vi "FestoCPX.Station.ProdSuctionGripper.Ready.vi"(7 "Log (T)":bool=TRUE, 8 "error in":errorcluster, 9 "Position":T1, 10 "Type":T2) -> (0 "error out":errorcluster, 2 "Ready state":T3)   [LabVIEW 2016]
uses:
  FestoCPX.Station.ProdSuctionGripper.ReadyState.ctl
  Station/Station.ProductSuctionGripper.Type.ctl
  Station/Station.ValvePosition.ctl
  tools/EventLog/EventLog.EventSource.ctl
  tools/Translator/Translator.Message.ctl
  tools/EventLog/EventLog.CreateError(array).vi
  tools/Translator/Translator.Translate.Status (NoError).vi
  tools/Translator/Translator.FormatMessage.vi
  tools/Translator/Translator.Global.vi
  tools/ErrorHandling/ErrorHandling.Create.vi
  Station/Station.Global.vi
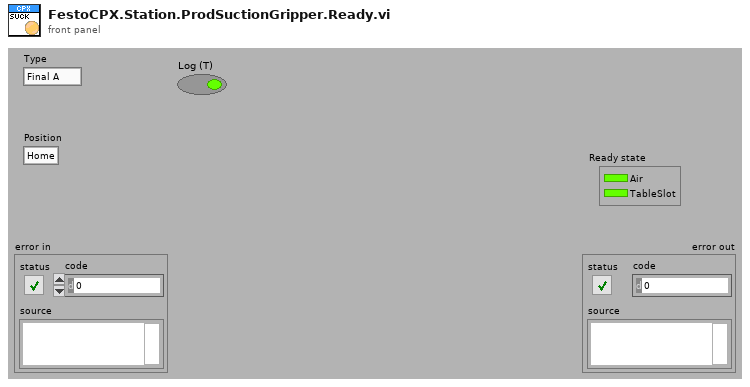
[diagram p1: front panel]
types:
  T1 = typedef "Station.ValvePosition.ctl" = enum16{"Home", "Work"}
  T2 = typedef "Station.ProductSuctionGripper.Type.ctl" = enum8{"Final A", "Final B", "Slot 1 A", "Slot 1 B", "Slot 2 A", "Slot 2 B", "Slot 3 A", "Slot 3 B", "Slot 4 A", "Slot 4 B"}
  T3 = typedef "FestoCPX.Station.ProdSuctionGripper.ReadyState.ctl" = cluster{"Air":bool, "TableSlot":bool}
  T4 = typedef "EventLog.EventSource.ctl" = enum16{"All", "Gui", "Ref", "File", "Arch", "Seq", "CPX", "DB", "Laser", "Scan.P", "Scan.O"}
  T5 = typedef "Translator.Message.ctl" = enum16{"-", "Event confirmed", "Log out", "Log in", "Shutdown", "Cancel", "Start", "Begin time", "End time", "Duration", "Service Mode", "Ignore Results", "Serial Format", "On", "Off", "OK", "NOK", "NOK %s", "Home", "Work", "Close", "Open", "In progress...", "Missing", "Empty", "Hardware failure", "Initial", "Default", "Total", "Out of range", "Free disk space is below 1GB - contact technician", "Error %d >> %s", "Error %d >> %s >> %s", "Msg %d >> %s", "Laser msg %d %s", "Laser cmd error %s %d", "Laser cmd failed %s", "Laser cmd warning %s", "Laser disconnected", "Laser status %s", "Laser already started", "Laser job unkonwn %s", "Laser job missing %s", "Laser job select failure %s", "Unable to start laser printing (%s)", "Unable to stop laser printing (%s)", "Laser marking aborted", "Laser marking timeout", "Unable to reset Laser Interlock (%s)", "Unable to trigger Laser. Laser not ready (%s)", "Laser job '%s' coordinates not configured", "Starting %s", "Quitting %s", "Configured", "Initializing", "Quitting", "Loading", "Loaded %d results", "Loaded %d events", "Running", "Stopped", "Summary", "Laser", "Do you want to continue?", "Do you want to delete the configuration?", "The configuration is being used by an order. Unable to delete!", "Press confirm button", "Station is not based. Do you want to exit?", "Station requires changeover. Do you want to run the test?", "Test options are not set as default. Do you want to continue?", "Formatting of WabcoNo is disabled. Do you want to continue?", "Product not detected. Do you want to continue?", "Product scan failed. Do you want to continue?", "Calibration", "Log out?", "System", "All", "IDLE", "Translating...%s", "Not found", "Alarm %s", "Run", "Skip", "Abort", "Repeat", "Please wait...", "Database disconnected", "Database disconnected - changeover disabled!", "Login to database successful", "Login to database failed: %d; %s", "Unable to check the product status of reference %d - database disconnected", "Unable to set the product status of reference %d - database disconnected", "Variant file backup %s", "Read variant (%s)", "Result", "Station armed!", "Station requires changeover!", "Select reference number...", "EMERGENCY BUTTON - press Control button", "EMERGENCY DOOR - press Control button", "Resetting Emergency...", "Unable to reset safety circuit - Emergency Button pressed", "Unable to reset safety circuit - Emergency Side Door open", "Station not based", "Station based", "Station not empty", "Station basing...", "No order", "Press Start to begin new order", "Scanning new order", "Order NOK. Correct or scan again", "Order OK. Press Accept", "Order ready", "Revolver incorrect", "Fork incorrect", "Revolver missing", "Revolver empty", "Container missing", "Offline results", "Offline statistics", "Updating statistics %.1f %%", "DMC Configurator", "Door open", "Close the front door", "Press start button", "Done. Open the front door", "Running...", "Running...%.1f %%", "Pause %s", "Pause %s. NOK container missing", "Pause %s. OK container missing", "Pause %s. Revolver empty", "Pause %s. Revolver missing", "Pause %s. Revolver incorrect", "Pause %s. Fork missing", "Pause %s. Fork incorrect", "Pause %s. Too many failures", "Pause %s. Unloading failure", "Pause %s. One slot is not working", "Pause %s. Part order is done. Empty OK container", "Pause %s. Unable to move product to slot", "Pause %s. Unable to move back product pusher", "Pause %s. Unable to lift product", "Pause %s. Unable to move back product lifter", "Pause %s. Unable to move product arm to Work", "Pause %s. Unable to move product arm to NOK", "Pause %s. Unable to move product arm to OK", "Pause %s. Unable to unsuck the NOK product", "Pause %s. Unable to drop the NOK product", "Pause %s. Product OK missing", "Pause %s. Unable to unsuck the OK product", "Pause %s. Unable to drop the OK product", "Stopping...", "File '%s' is missing", "File '%s' is broken", "File '%s' is running", "Log file started (%s)", "Log file ended (%s)", "Log file stopped (%s)", "Log file ignored (%s)", "Log file exported (%s)", "Log file export failed (%s)", "Wrong serial number in log file", "Wrong reference number in log file", "Test steps are missing", "%s = %.3f", "Process param '%s' not found in DB", "Process param '%s' wrong order", "Process param '%s' value %.3f out of limits (%.3f; %.3f)", "Step%d param '%s' not found in DB", "Step%d param '%s' wrong order", "Step%d param '%s' value %.3f out of limits (%.3f; %.3f)", "Step%d EV '%s' not found in DB", "Step%d EV '%s' wrong order", "\"%s\" not found in DB", "\"%s\" wrong order", "\"%s\" value %.3f out of limits (%.3f; %.3f)", "\"%s\" not found in software", "Process init (%s)", "Process started", "Process restarted", "Process run", "Process done", "Process done - remove OK container", "Process aborted", "Process aborted at work", "Process aborted at home", "Process error", "Process error at home", "Process error at work", "Process close", "Process pause", "Process continue", "Process door open", "Process door close", "Process pause at slot %s due to %s", "Select plate from the order to process", "Do you want to start the process?", "Do you want to continue the process?", "There is unfinished order. Do you want to put the new order?", "Product %s %d OK", "Product %s %d NOK", "Unable to unload the slot %s. Product missing in the slot", "Unable to unload the slot %s. Product already in the arm", "Unable to accept the product as OK. Product missing in slot %s", "Unable to accept the product as OK. Product could not drop into the container at slot %s", "Unable to accept the product as NOK. Product could not drop into the container at slot %s", "Scan failed. Error %s", "Scan failed. Scanner disconnected", "Scan failed. Wrong Wabco number %d, limit (%d,%d)", "Scan failed. Wrong serial number %d, limit (%d,%d)", "Scan failed. Wrong date %d, limit (%d,%d)", "Scan failed. Wrong product wabco number %d (expected %d)", "Scan failed. Wrong product serial number %d (expected > 0)", "Scan OK %s", "Scan failed. Unable to determine table position (%s)", "Scan failed. Timeout", "Tune failed. Scanner disconnected", "Tune failed. Timeout", "%s = %d", "%s = %d->%d", "Unable to set %s = %.2f - Air Pressure Inside off", "Unable to set digital output '%s' = %d", "Unable to activate air pressure inside - timeout", "Unable to activate air pressure inside - aborted", "Unable to switch on Air Main Valve - Air Pressure Inlet off", "Unable to switch on Air Main Valve - Door open", "Unable to switch off Air Main Valve - timeout", "Unable to switch off Air Main Valve - aborted", "Unable to rotate Table - timeout", "Unable to rotate Table - aborted", "Unable to rotate Table - Product Move not in Home position", "Unable to rotate Table - Air Pressure Inside off", "Unable to rotate Table - Product Lift A not in Home position", "Unable to rotate Table - Product Lift B not in Home position", "Unable to rotate Table - unlock before movement timeout", "Unable to rotate Table - lock after movement timeout", "Unable to move Table Lock to %s position - timeout", "Unable to move Table Lock to %s position - aborted", "Unable to move Table Lock to %s position - Air Pressure Inside off", "Unable to move Table Lock to %s position - Table not in position", "Unable to move Product Lift A to %s position - timeout", "Unable to move Product Lift B to %s position - timeout", "Unable to move Product Lift A to %s position - aborted", "Unable to move Product Lift B to %s position - aborted", "Unable to move Product Lift A to %s position - Air Pressure Inside off", "Unable to move Product Lift B to %s position - Air Pressure Inside off", "Unable to move Product Lift A to %s position - Table not locked", "Unable to move Product Lift B to %s position - Table not locked", "Unable to move Product Lift A to %s position - Product Arm not in Work position", "Unable to move Product Lift B to %s position - Product Arm not in Work position", "Unable to set Product Suction Gripper %s to %s - timeout", "Unable to set Product Suction Gripper %s to %s - aborted", "Unable to set Product Suction Gripper %s to %s - Air Pressure Inside off", "Unable to set Product Suction Gripper %s to %s - Table slot unkown", "Unable to move Product Arm to %s position - timeout", "Unable to move Product Arm to %s position - aborted", "Unable to move Product Arm to %s position - Air Pressure Inside off", "Unable to move Product Arm to %s position - Product Lift A not in Home position", "Unable to move Product Arm to %s position - Product Lift B not in Home position", "Unable to move Product to %s position - timeout", "Unable to move Product to %s position - aborted", "Unable to move Product to %s position - Air Pressure Inside off", "Unable to move Product to %s position - Table not in position"}
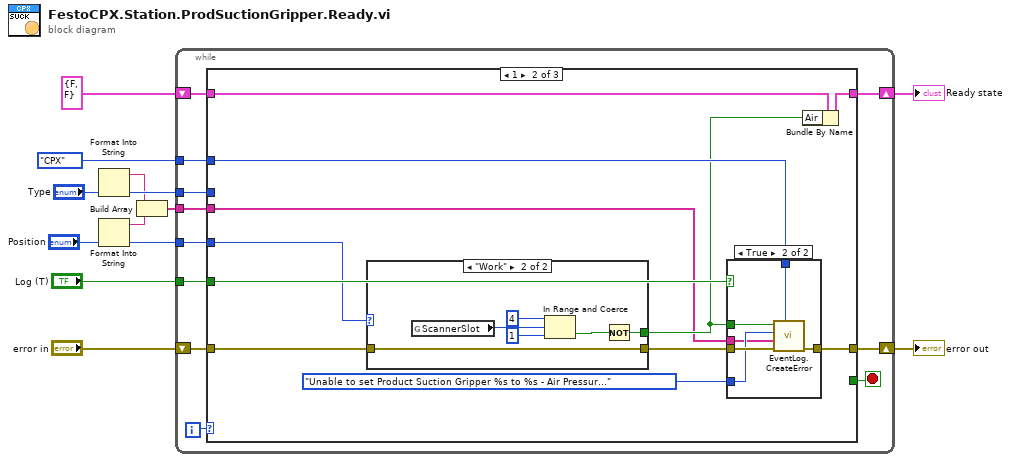
[diagram p0: block diagram]
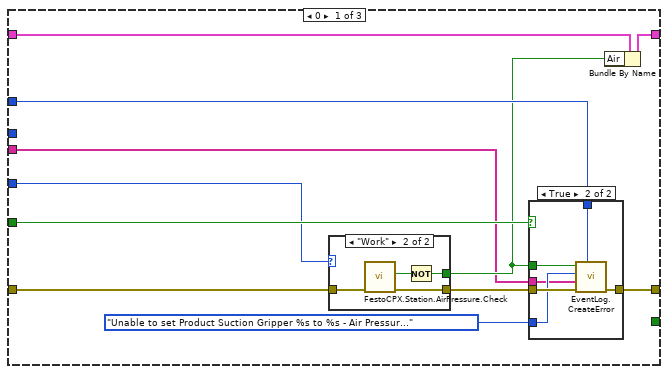
[diagram p2: hidden frame]
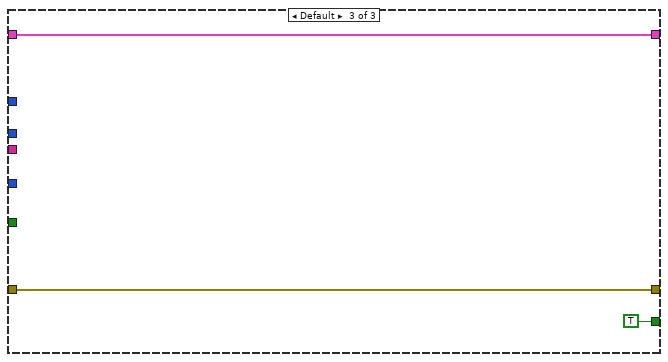
[diagram p7: hidden frame]
diagram:
  n1 = Format Into String("Type") -> (resulting string=w3:string)  [unwired: 3 in, 1 out]
  n2 = Format Into String("Position") -> (resulting string=w2:string)  [unwired: 3 in, 1 out]
  n3 = Build Array(w3, w2) -> (w1:string[])
  n4 = while {
    tunnel: "Log (T)" -> [w21]
    tunnel: EventLog.EventSource."CPX" ("Source") -> [w20]
    shift-right: [w15] -> w8
    shift-left: "error in" -> [w22]
    shift-right: [w16] -> w6
    shift-left: T3 {"Air"=FALSE, "TableSlot"=FALSE} ("Ready state") -> [w17]
    tunnel: "Type" -> [w14]
    tunnel: "Position" -> [w13]
    tunnel: w1 -> [w12]
    i -> [w19]
    stop <- w18 stop-if-true
    n5 = case shown="1" w19 {
      tunnel: w22 -> [w23 w46 w72]
      tunnel: [w28 w51 w71] -> w16
      tunnel: w21 -> [w27 w50 _]
      tunnel: w20 -> [w30 w53 _]
      tunnel: [_ _ TRUE] -> w18
      tunnel: w17 -> [w29 w52 w71]
      tunnel: [w31 w54 w72] -> w15
      tunnel: w14 -> [_ _ _]
      tunnel: w13 -> [w25 w48 _]
      tunnel: w12 -> [w24 w47 _]
      frame 0 {
        n6 = case shown="\"Work\"" w25 {
          tunnel: [w34 w38] -> w33
          tunnel: [_ w36] -> w26
          tunnel: w23 -> [w34 w37]
          frame "Home" {
          }
          frame "Work" {
            n7 = call "FestoCPX.Station.AirPressure.Check.vi"("error in"=w37) -> ("error out"=w38:errorcluster, "Air pressure Inside"=w35:bool)  [unwired: 7 in, 2 out]
            n8 = Not(x=w35) -> (.not. x?=w36:bool)
          }
        }
        n9 = case shown="True" w27 {
          tunnel: w30 -> [_ w45]
          tunnel: w26 -> [_ w44]
          tunnel: w33 -> [w39 w43]
          tunnel: Translator.Message."Unable to set Product Suction Gripper %s to %s - Air Pressure Inside off" ("msg") -> [_ w42]
          tunnel: [w39 w41] -> w31
          tunnel: w24 -> [_ w40]
          frame False {
          }
          frame True {
            n10 = call-poly "EventLog.CreateError.vi"("Source (All)"=w45, "error in"=w43, "args"=w40, "msg"=w42, "create (T)"=w44) -> ("error out"=w41:errorcluster)  [unwired: 5 in, 1 out]
          }
        }
        n11 = Bundle By Name(cluster=w29, "Air"=w26) -> (w28:T3)
      }
      frame 1 {
        n12 = case shown="\"Work\"" w48 {
          tunnel: [w57 w58] -> w56
          tunnel: [_ w63] -> w49
          tunnel: w46 -> [w57 w58]
          frame "Home" {
          }
          frame "Work" {
            n13 = global read "Station.Global.vi" "ScannerSlot"() -> (w60:i32)
            n14 = In Range and Coerce(upper limit=4, x=w60, lower limit=1) -> (In Range?=w59:bool)  [unwired: 1 out]
            n15 = Not(x=w59) -> (.not. x?=w63:bool)
          }
        }
        n16 = case shown="True" w50 {
          tunnel: w53 -> [_ w70]
          tunnel: w49 -> [_ w69]
          tunnel: w56 -> [w64 w68]
          tunnel: Translator.Message."Unable to set Product Suction Gripper %s to %s - Air Pressure Inside off" ("msg") -> [_ w67]
          tunnel: [w64 w66] -> w54
          tunnel: w47 -> [_ w65]
          frame False {
          }
          frame True {
            n17 = call-poly "EventLog.CreateError.vi"("Source (All)"=w70, "error in"=w68, "args"=w65, "msg"=w67, "create (T)"=w69) -> ("error out"=w66:errorcluster)  [unwired: 5 in, 1 out]
          }
        }
        n18 = Bundle By Name(cluster=w52, "Air"=w49) -> (w51:T3)
      }
      frame Default {
      }
    }
  }
  "error out" <- w8
  "Ready state" <- w6
